vi "SaveSettings.vi"(0 "object in":refnum<class "Experiment2.lvclass">, 5 "error in (no error)":errorcluster) -> (14 "object out":refnum<class "Experiment2.lvclass">, 19 "error out":errorcluster)   [LabVIEW 2024, in "Experiment2.lvclass"]
uses:
  Experiment2.lvclass
  Experiment2.lvclass/Experiment2.ctl
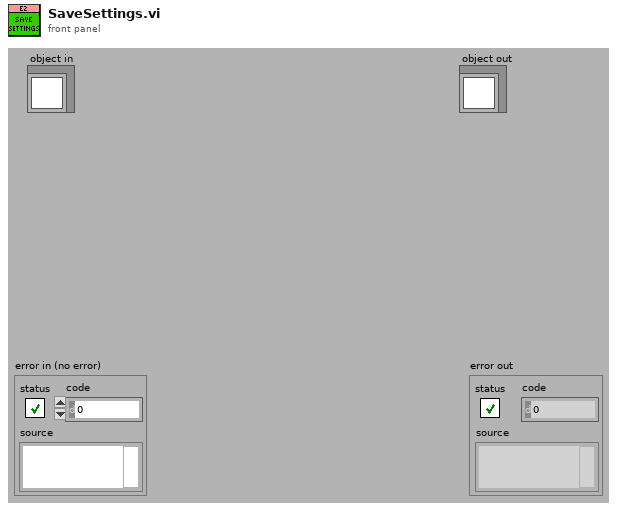
[diagram p1: front panel]
types:
  T1 = typedef "AD2_WFG_SDK.lvclass/WFG.ctl" = cluster{"Running":bool, "Ch1":T2, "Ch2":T2, "SyncronizeState":enum16{"Independent", "Ch1Master", "Ch2Master"}}
  T2 = typedef "AD2_WFG_SDK.lvclass/WFGCh.ctl" = cluster{"idxChannel":i32, "Settings out of range":bool, "Carrier":cluster{"Frequency (Hz)":dbl, "Amplitude (V)":dbl, "Offset(V)":dbl, "Symmetry(%) ":dbl, "Phase(Deg)":dbl, "Function":u16, "Enable":bool}, "Trigger":cluster{"secRun(0=Cont)":dbl, "secWait":dbl, "cRepeat(0=inf)":i32, "Repeat Trigger":bool, "TrigrSrc":T3}, "FM Mod":cluster{"Frequency (Hz)":dbl, "Amplitude (%)":dbl, "Offset(V)":dbl, "Symmetry(%) ":dbl, "Phase(Deg)":dbl, "Function 2":u16, "Enable":bool}}
  T3 = typedef "AD2_SDK.lvclass/AD2TriggerSources.ctl" = enum8{"trigrsrcNone", "trigsrcPC", "trigsrcDetectorAnalogIn", "trigsrcDetectorDigitalIn", "trigsrcAnalogIn", "trigsrcDigitalIn", "trigsrcDigitalOut", "trigsrcAnalogOut1", "trigsrcAnalogOut2", "trigsrcAnalogOut3", "trigsrcAnalogOut4", "trigsrcExternal1", "trigsrcExternal2", "trigsrcExternal3", "trigsrcExternal4", ""}
  T4 = typedef "AD2_DO_SDK.lvclass/DOTrigger.ctl" = cluster{"secRun(0=Cont)":dbl, "secWait":dbl, "cRepeat(0=inf)":i32, "Repeat Trigger":bool, "TrigrSrc":T3}
  T5 = cluster{"DO Trigger":T4, "ClockSettings":cluster{"Frequency":dbl, "Enable":bool, "IdleState":enum16{"Initial", "Low", "High", "Z"}}[]}
  T6 = cluster{"Master Pulse Settings":cluster{"Mode":u32, "Source":u32, "Interval":dbl, "Burst":u32}, "Capture mode":i32, "Frames":i32, "Dcam Trigger Source":i32, "External Options":cluster{"Polarity":i32, "Delay":dbl}, "ExposureTime(ms)":dbl}
  T7 = cluster{"Flush Flowrate":dbl, "flush volume (ul)":dbl, "WaitAfterFlush":dbl}
  T8 = cluster{"Frequency":dbl, "Enable":bool, "IdleState":enum16{"Initial", "Low", "High", "Z"}}[]
  T9 = cluster{"Frequency":dbl, "Enable":bool, "IdleState":enum16{"Initial", "Low", "High", "Z"}}
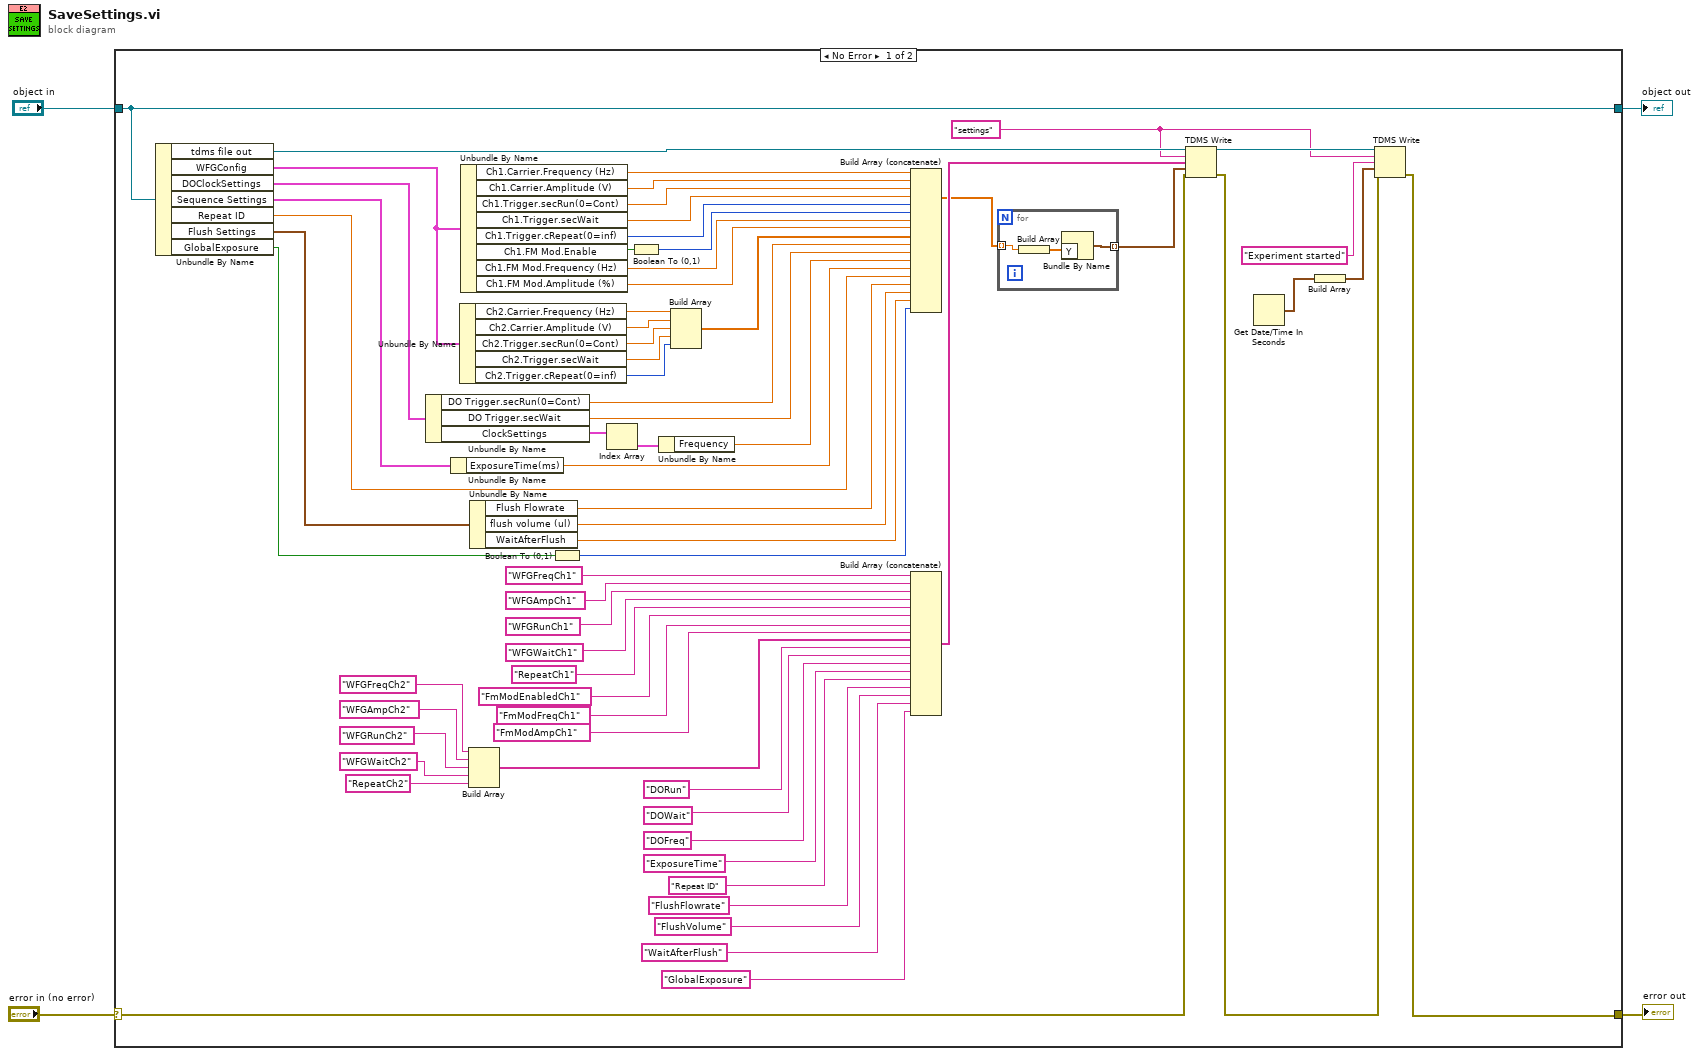
[diagram p0: block diagram]
diagram:
  n1 = case shown="No Error" "error in (no error)" {
    selector: "error in (no error)" -> [w69 w76]
    tunnel: [w22 w76] -> w3
    tunnel: [w71 w75] -> w1
    tunnel: "object in" -> [w71 w75]
    frame No Error {
      w45 = "settings" ("group name in (Untitled)")
      n2 = Unbundle By Name(w71) -> ("tdms file out"=w70:refnum<k34>, "WFGConfig"=w36:T1, "DOClockSettings"=w68:T5, "Sequence Settings"=w67:T6, "Repeat ID"=w49:dbl, "Flush Settings"=w21:T7, "GlobalExposure"=w14:bool)
      n3 = Unbundle By Name(w68) -> ("DO Trigger.secRun(0=Cont)"=w53:dbl, "DO Trigger.secWait"=w52:dbl, "ClockSettings"=w41:T8)
      n4 = Unbundle By Name(w67) -> ("ExposureTime(ms)"=w39:dbl)
      n5 = Unbundle By Name(w36) -> ("Ch2.Carrier.Frequency (Hz)"=w35:dbl, "Ch2.Carrier.Amplitude (V)"=w34:dbl, "Ch2.Trigger.secRun(0=Cont)"=w33:dbl, "Ch2.Trigger.secWait"=w32:dbl, "Ch2.Trigger.cRepeat(0=inf)"=w31:i32)
      n6 = Unbundle By Name(w36) -> ("Ch1.Carrier.Frequency (Hz)"=w59:dbl, "Ch1.Carrier.Amplitude (V)"=w58:dbl, "Ch1.Trigger.secRun(0=Cont)"=w57:dbl, "Ch1.Trigger.secWait"=w56:dbl, "Ch1.Trigger.cRepeat(0=inf)"=w54:i32, "Ch1.FM Mod.Enable"=w10:bool, "Ch1.FM Mod.Frequency (Hz)"=w8:dbl, "Ch1.FM Mod.Amplitude (%)"=w6:dbl)
      n7 = Build Array("WFGFreqCh2" ("group name in (Untitled)"), "WFGAmpCh2" ("group name in (Untitled)"), "WFGRunCh2" ("group name in (Untitled)"), "WFGWaitCh2" ("group name in (Untitled)"), "RepeatCh2" ("group name in (Untitled)")) -> (w24:string[])
      n8 = Unbundle By Name(w21) -> ("Flush Flowrate"=w18:dbl, "flush volume (ul)"=w17:dbl, "WaitAfterFlush"=w16:dbl)
      n9 = Boolean To (0,1)(Boolean=w14) -> (0, 1=w13:i16)
      n10 = Index Array(array=w41) -> (element=w40:T9)  [unwired: 1 in]
      n11 = Boolean To (0,1)(Boolean=w10) -> (0, 1=w9:i16)
      n12 = Unbundle By Name(w40) -> ("Frequency"=w38:dbl)
      n13 = Build Array(w35, w34, w33, w32, w31) -> (w30:dbl[])
      n14 = Build Array (concatenate)(w59, w58, w57, w56, w54, w9, w8, w6, w30, w53, w52, w38, w39, w49, w18, w17, w16, w13) -> (w48:dbl[])
      n15 = Build Array (concatenate)("WFGFreqCh1" ("group name in (Untitled)"), "WFGAmpCh1" ("group name in (Untitled)"), "WFGRunCh1" ("group name in (Untitled)"), "WFGWaitCh1" ("group name in (Untitled)"), "RepeatCh1" ("group name in (Untitled)"), "FmModEnabledCh1" ("group name in (Untitled)"), "FmModFreqCh1" ("group name in (Untitled)"), "FmModAmpCh1" ("group name in (Untitled)"), w24, "DORun" ("group name in (Untitled)"), "DOWait" ("group name in (Untitled)"), "DOFreq" ("group name in (Untitled)"), "ExposureTime" ("group name in (Untitled)"), "Repeat ID" ("group name in (Untitled)"), "FlushFlowrate" ("group name in (Untitled)"), "FlushVolume" ("group name in (Untitled)"), "WaitAfterFlush" ("group name in (Untitled)"), "GlobalExposure" ("group name in (Untitled)")) -> (w51:string[])
      n16 = for {
        tunnel: w48 -> [w74] mode=indexing
        tunnel: [w72] -> w47 mode=indexing
        n17 = Build Array(w74) -> (w73:dbl[])
        n18 = Bundle By Name("Y"=w73) -> (w72:waveform(dbl))  [unwired: 1 in]
      }
      n19 = TDMS Write(0:w70, 5:w45, 7:w51, 9:w47, 11:w69) -> (4:w46:refnum<k34>, 15:w23:errorcluster)  [unwired: 1 in, 2 out]
      n20 = Get Date/Time In Seconds() -> (seconds since 1Jan1904=w43:timestamp)
      n21 = Build Array(w43) -> (w42:timestamp[])
      n22 = TDMS Write(0:w46, 5:w45, 7:"Experiment started" ("group name in (Untitled)"), 9:w42, 11:w23) -> (15:w22:errorcluster)  [unwired: 1 in, 3 out]
    }
    frame Error {
    }
  }
  "error out" <- w3
  "object out" <- w1
